vi "Evalmutlivar.vi"(2 "error in (no error)":errorcluster, 3 "Variables":string[](array[string])=["Vxx", "Vxy", "DMM I", "DMM V"], 4 "Matrix data":dbl[][](array[numeric]), 5 "formula":string) -> (0 "error out":errorcluster, 1 "Y Values":dbl[](array[numeric]) format="%.2f")   [LabVIEW 2011]
uses:
  <vilib>/gmath/NI_Gmath.lvlib
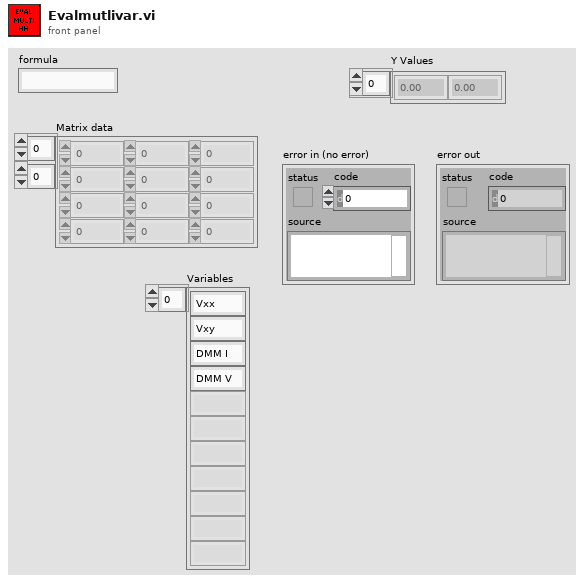
[diagram p1: front panel]
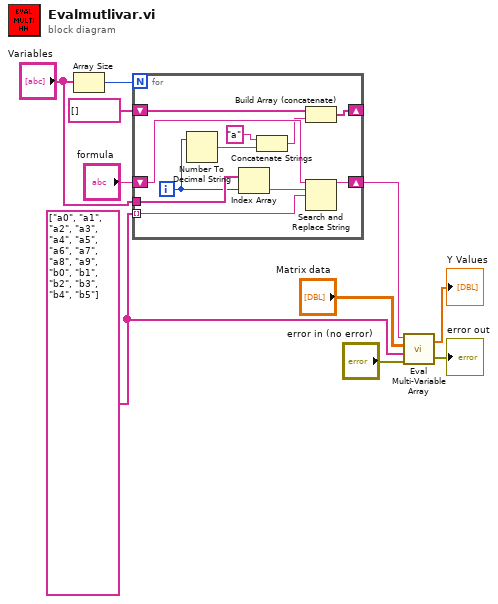
[diagram p0: block diagram]
diagram:
  w2 = string[] ["a0", "a1", "a2", "a3", "a4", "a5", "a6", "a7", "a8", "a9", "b0", "b1", "b2", "b3", "b4", "b5"] ("Variables")
  n1 = Array Size(array="Variables") -> (size(s)=w9:i32)
  n2 = for {
    N: w9 -> [_]
    tunnel: "Variables" -> [w21]
    shift-right: [w19] -> w6
    shift-left: "formula" -> [w20]
    shift-right: [w12] -> _
    shift-left: string[] [] ("Variables") -> [w13]
    tunnel: w2 -> [w11] mode=indexing
    i -> [w18]
    n3 = Number To Decimal String(number=w18) -> (decimal integer string=w17:string)  [unwired: 1 out]
    n4 = Index Array(array=w21, index=w18) -> (element=w15:string)
    n5 = Concatenate Strings("a", w17) -> (w14:string)
    n6 = Build Array (concatenate)(w13, w14) -> (w12:string[])
    n7 = Search and Replace String(input string=w20, search string=w15, replace string=w11) -> (result string=w19:string)  [unwired: 2 in, 6 out]
  }
  n8 = call <vilib>:"Eval Multi-Variable Array.vi"("error in (no error)"="error in (no error)", "Variables"=w2, "X Values"="Matrix data", "formula"=w6) -> ("error out"=→"error out":errorcluster, "Y Values"=→"Y Values":dbl[])
